vi "数据上传-15.vi"(1 "完成时间":string, 2 "打标内容":string, 3 "打标机合格":bool, 4 "操作者":string, 5 "产品ID":string) -> ()   [LabVIEW 2013]
uses:
  <vilib>/Utility/error.llb/whitespace.ctl
panel:
  in  "error in (no error)":errorcluster
  out "error out":errorcluster
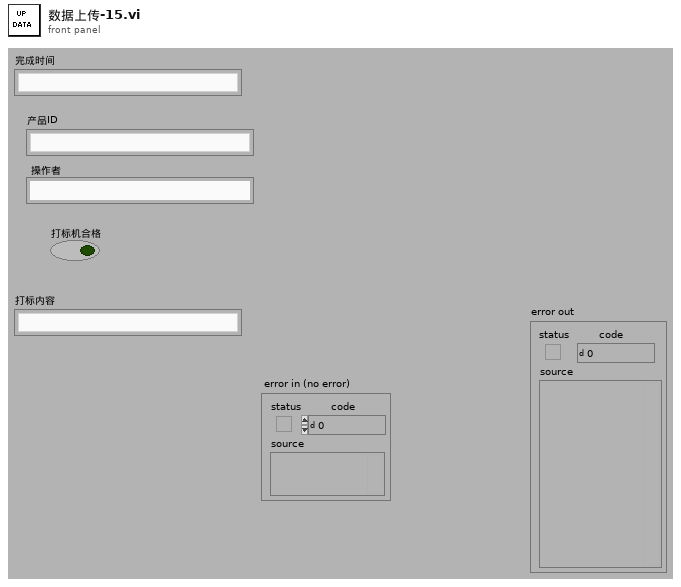
[diagram p1: front panel]
types:
  T1 = typedef "whitespace.ctl" = u16
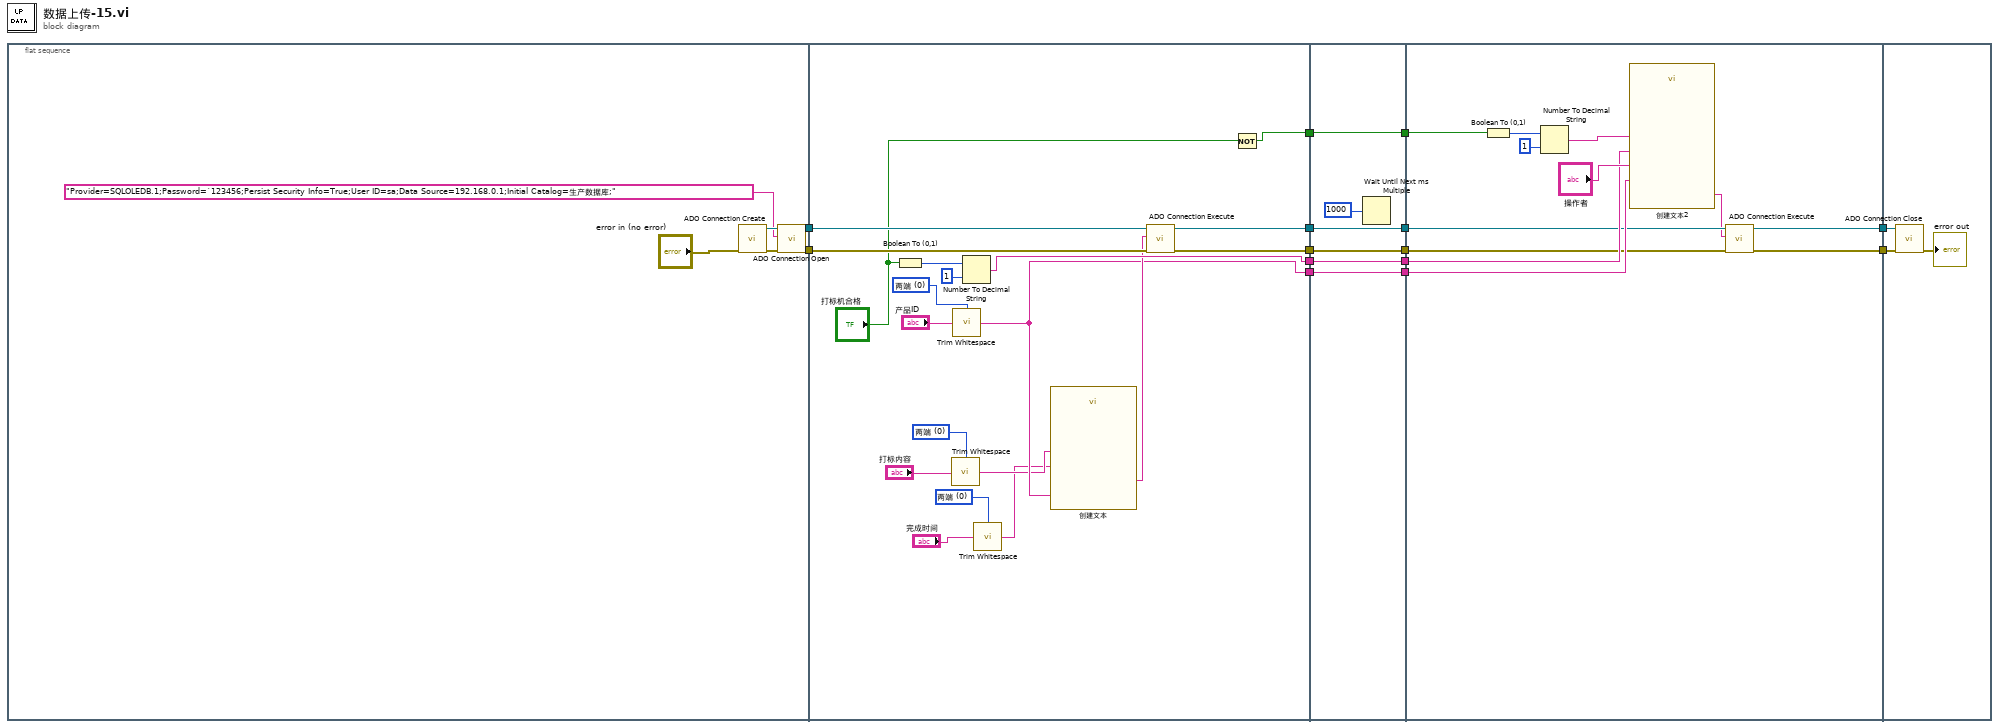
[diagram p0: block diagram]
diagram:
  n1 = flat-sequence {
    tunnel: [w16] -> w14
    tunnel: [w17] -> w13
    tunnel: w14 -> [w39]
    tunnel: w13 -> [w38]
    tunnel: [w37] -> w12
    tunnel: [w35] -> w10
    tunnel: [w32] -> w8
    tunnel: [w25] -> w6
    tunnel: [w30] -> w1
    tunnel: w12 -> [w45]
    tunnel: [w45] -> w11
    tunnel: w10 -> [w44]
    tunnel: [w44] -> w9
    tunnel: w8 -> [w43]
    tunnel: [w43] -> w7
    tunnel: w6 -> [w42]
    tunnel: [w42] -> w5
    tunnel: [w40] -> w2
    tunnel: w1 -> [w40]
    tunnel: w11 -> [w51]
    tunnel: w9 -> [w50]
    tunnel: w7 -> [w53]
    tunnel: w5 -> [w52]
    tunnel: [w48] -> w4
    tunnel: [w47] -> w3
    tunnel: w2 -> [w46]
    tunnel: w4 -> [w59]
    tunnel: w3 -> [w58]
    frame #0 {
      n2 = call "ADO Connection Create.vi"("error in (no error)"="error in (no error)") -> ("error out"=w19:errorcluster, "ADODB._Connection Out"=w18:refnum<k7>)  [unwired: 9 out]
      n3 = call "ADO Connection Open.vi"("error in (no error)"=w19, "ConnectionString"="Provider=SQLOLEDB.1;Password=`123456;Persist Security Info=True;User ID=sa;Data Source=192.168.0.1;Initial Catalog=生产数据库;" ("字符串 2"), "ADODB._Connection In"=w18) -> ("error out"=w16:errorcluster, "ADODB._Connection Out"=w17:refnum<k7>)  [unwired: 7 out]
    }
    frame #1 {
      w23 = T1 0 items=["两端", "字符串首端", "字符串末端"] ("location (both)")
      w28 = T1 0 items=["两端", "字符串首端", "字符串末端"] ("location (both)")
      w36 = T1 0 items=["两端", "字符串首端", "字符串末端"] ("location (both)")
      n4 = Boolean To (0,1)(Boolean="打标机合格") -> (0, 1=w34:i16)
      n5 = call <vilib>:"Trim Whitespace.vi"("string"="打标内容", "location (both)"=w28) -> ("trimmed string"=w24:string)
      n6 = call <vilib>:"Trim Whitespace.vi"("string"="产品ID", "location (both)"=w36) -> ("trimmed string"=w25:string)
      n7 = Number To Decimal String(number=w34, width (-)=i16 1 ("宽度(-)")) -> (decimal integer string=w32:string)
      n8 = call <vilib>:"Trim Whitespace.vi"("string"="完成时间", "location (both)"=w23) -> ("trimmed string"=w21:string)
      n9 = call "创建文本"("完成时间"=w21, "打标内容"=w24, "产品ID"=w25) -> ("Result"=w26:string)  [unwired: 11 in, 1 out]
      n10 = call "ADO Connection Execute.vi"("error in (no error)"=w39, "CommandText"=w26, "ADODB._Connection In"=w38) -> ("error out"=w35:errorcluster, "ADODB._Connection Out"=w37:refnum<k7>)  [unwired: 7 out]
      n11 = Not(x="打标机合格") -> (.not. x?=w30:bool)
    }
    frame #2 {
      n12 = Wait Until Next ms Multiple(millisecond multiple=u32 1000 ("毫秒倍数")) -> ()  [unwired: 1 out]
    }
    frame #3 {
      n13 = Boolean To (0,1)(Boolean=w46) -> (0, 1=w54:i16)
      n14 = Number To Decimal String(number=w54, width (-)=i16 1 ("宽度(-)")) -> (decimal integer string=w56:string)
      n15 = call "创建文本2"("产品ID"=w52, "操作者"="操作者", "本序不合格"=w56, "本序合格"=w53) -> ("Result"=w49:string)  [unwired: 10 in, 1 out]
      n16 = call "ADO Connection Execute.vi"("error in (no error)"=w50, "CommandText"=w49, "ADODB._Connection In"=w51) -> ("error out"=w47:errorcluster, "ADODB._Connection Out"=w48:refnum<k7>)  [unwired: 7 out]
    }
    frame #4 {
      n17 = call "ADO Connection Close.vi"("error in (no error)"=w58, "ADODB._Connection In"=w59) -> ("error out"=→"error out":errorcluster)  [unwired: 9 out]
    }
  }
